vi "main.vi"() -> ()   [LabVIEW 2020]
panel:
  out "Códigos Encontrados":string[](array[string])
  in  "Image Path":path=path "E:/GitHub/Etiquetas-com-API/Fotos teste/IMG_20210329_182819.jpg"
  in  "Fonte das imagens":enum16{"Câmera", "Imagens na pasta"}(ring)
  in  "Stop (F)":bool
  out "Image Out":T1(plugin-control)
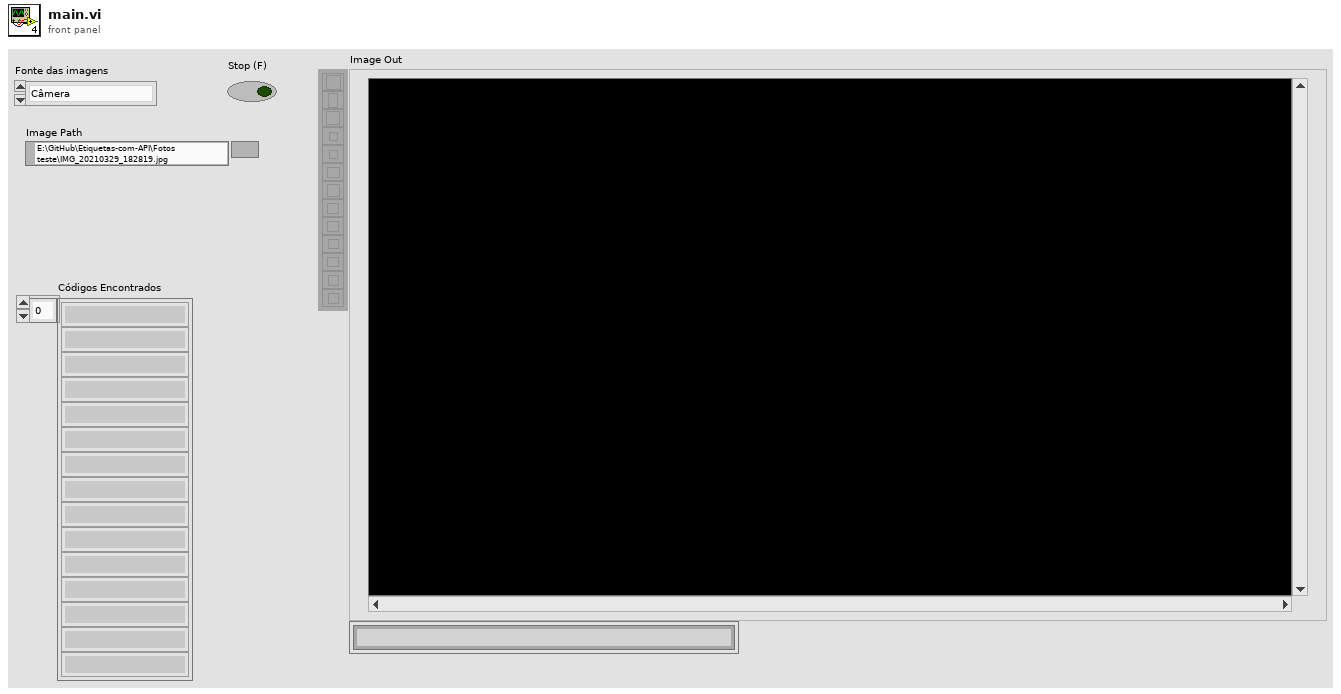
[diagram p1: front panel]
types:
  T1 = typedef "IMAQ Image.ctl" = refnum<image>
  T2 = cluster{"Data":string, "Special Char 1":string, "Special Char 2":string, "Checksum(s)":string, "Barcode Type":u32, "Confidence Level":sgl, "Bounding Box":cluster{"x":sgl, "y":sgl}[]}[]
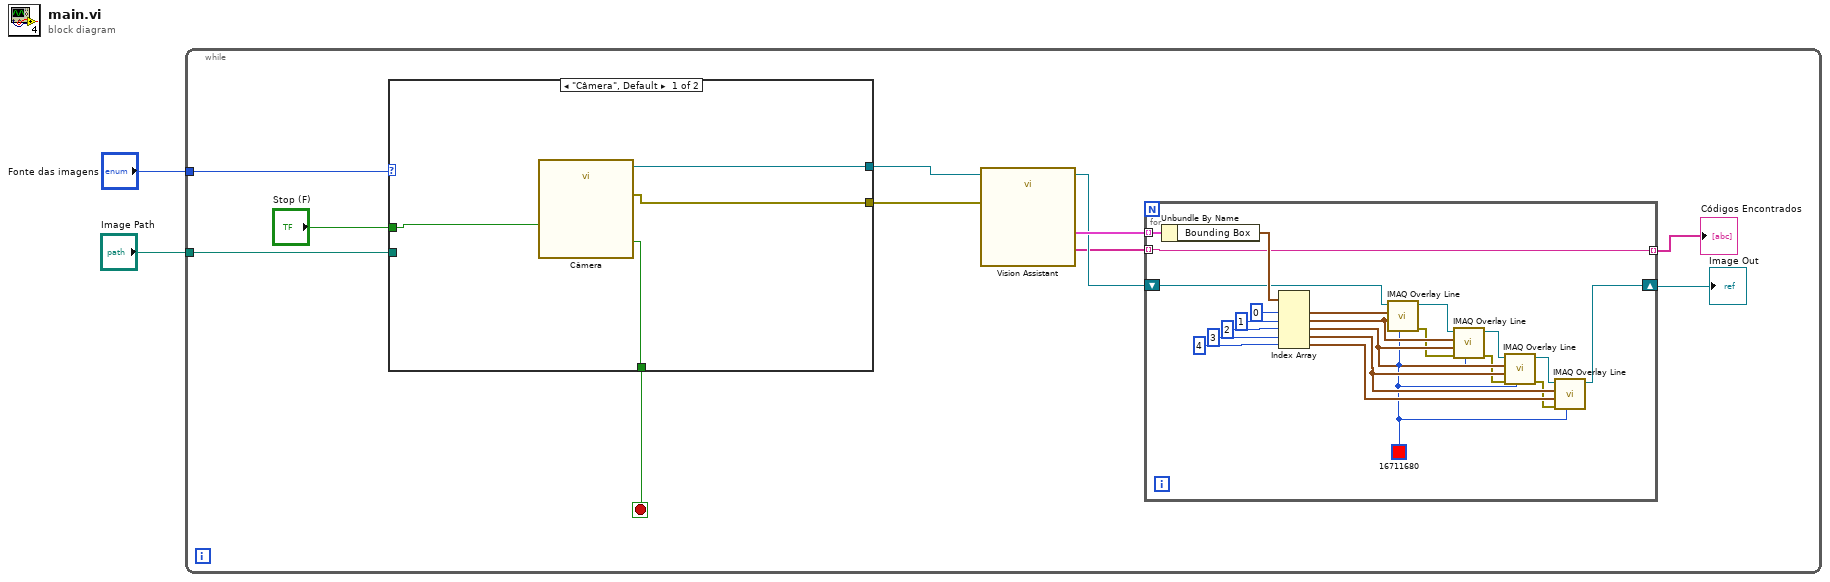
[diagram p0: block diagram]
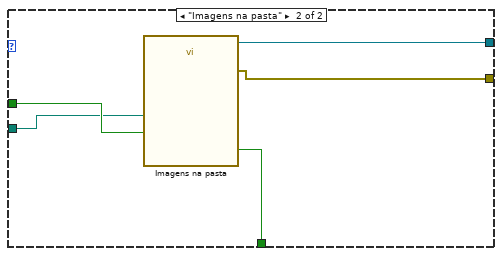
[diagram p2: hidden frame]
diagram:
  n1 = while {
    tunnel: "Fonte das imagens" -> [w11]
    tunnel: "Image Path" -> [w8]
    stop <- w12 stop-if-true
    n2 = case shown="\"Câmera\", Default" w11 {
      tunnel: "Stop (F)" -> [w39 w44]
      tunnel: [w37 w43] -> w10
      tunnel: [w38 w42] -> w12
      tunnel: [w36 w41] -> w9
      tunnel: w8 -> [_ w40]
      frame "Câmera", Default {
        n3 = call "Câmera"("Stop (F)"=w39) -> ("Image Out"=w37:T1, "Stopped"=w38:bool, "error out"=w36:errorcluster)  [unwired: 24 in]
      }
      frame "Imagens na pasta" {
        n4 = call "Imagens na pasta"("Image Path"=w40, "Stop (F)"=w44) -> ("Image Out"=w43:T1, "Stopped"=w42:bool, "error out"=w41:errorcluster)  [unwired: 23 in]
      }
    }
    n5 = call "Vision Assistant"("Image In"=w10, "error in"=w9) -> ("Image Out"=w6:T1, "Barcodes (Barcode Reader 1)"=w7:T2, "Complete Data (Barcode Reader 1)"=w4:string[])  [unwired: 22 in, 1 out]
    n6 = for {
      tunnel: w7 -> [w35] mode=indexing
      shift-right: [w15] -> w5
      shift-left: w6 -> [w16]
      tunnel: w4 -> [w14] mode=indexing
      tunnel: [w14] -> w3 mode=indexing
      w17 = u32 16711680 ("Color")
      n7 = Unbundle By Name(w35) -> ("Bounding Box"=w34:cluster{"x":sgl, "y":sgl}[])
      n8 = Index Array(array=w34, index #1=0 ("index"), index #2=1 ("index"), index #3=2 ("index"), index #4=3 ("index"), index #5=4 ("index")) -> (element #1=w28:cluster{"x":sgl, "y":sgl}, element #2=w27:cluster{"x":sgl, "y":sgl}, element #3=w26:cluster{"x":sgl, "y":sgl}, element #4=w25:cluster{"x":sgl, "y":sgl}, element #5=w24:cluster{"x":sgl, "y":sgl})
      n9 = call "IMAQ Overlay Line"("Color"=w17, "End Point"=w27, "Start Point"=w28, "Image"=w16) -> ("error out"=w23:errorcluster, "Image Out"=w18:T1)  [unwired: 6 in]
      n10 = call "IMAQ Overlay Line"("Color"=w17, "error in (no error)"=w23, "End Point"=w26, "Start Point"=w27, "Image"=w18) -> ("error out"=w22:errorcluster, "Image Out"=w19:T1)  [unwired: 5 in]
      n11 = call "IMAQ Overlay Line"("Color"=w17, "error in (no error)"=w22, "End Point"=w25, "Start Point"=w26, "Image"=w19) -> ("error out"=w21:errorcluster, "Image Out"=w20:T1)  [unwired: 5 in]
      n12 = call "IMAQ Overlay Line"("Color"=w17, "error in (no error)"=w21, "End Point"=w24, "Start Point"=w25, "Image"=w20) -> ("Image Out"=w15:T1)  [unwired: 5 in, 1 out]
    }
    "Image Out" <- w5
    "Códigos Encontrados" <- w3
  }
